vi "MF-101 I2C loopback dongle with command control and selectable output value.vi"() -> ()   [LabVIEW 8.6]
uses:
  <libdir>/resource/objmgr/ueidaq.rc
  vi.lib/UeiDaq/UeiDaqConfigureTimingForMessagingIO.vi
  vi.lib/UeiDaq/UeiDaqCreateI2CSlaveSession.vi
  vi.lib/UeiDaq/UeiDaqCreateI2CMasterSession.vi
panel:
  in  "Bus Monitor ACK":i32[](array[ring]) items=["Disabled", "Enabled"]
  in  "Bus Monitor":i32[](array[ring]) items=["Disabled", "Enabled"]
  in  "Termination":i32[](array[ring]) items=["Disabled", "Enabled"]
  in  "Loopback":i32[](array[ring]) items=["None", "Relay", "FPGA"]
  out "Bus Monitor ACK":i32[](array[ring]) items=["Disabled", "Enabled"]
  out "Bus Monitor":i32[](array[ring]) items=["Disabled", "Enabled"]
  out "Loopback":i32[](array[ring]) items=["None", "Relay", "FPGA"]
  out "AddressWidth":i32[](array[ring]) items=["7-bit", "10-bit"]
  in  "Slave Resource":string
  out "Termination":i32[](array[ring]) items=["750 Ohm", "1.5 kOhm"]
  in  "output value":u16
  in  "Message Size":i32
  out "Slave Read Data String":string
  out "Master Read Data String":string
  out "Slave Read Count":i32
  out "Master Read Count":i32
  in  "Command Type":u32(ring) items=["Write", "Read", "WriteRead"]
  out "Slave Tx Data":u16[](array[numeric]) format="%x"
  out "Slave Channel":i32
  out "Master Channel":i32
  in  "Stop":bool
  in  "Slave Address":i32
  in  "Slave Address Width":u32(ring) items=["7-bit", "10-bit"]
  in  "Bit Rate":i32(ring) items=["100kBitsPerSecond", "400kBitsPerSecond", "1MBitsPerSecond"]
  in  "TTL Level":i32(ring) items=["3.3V", "5V"]
  in  "Secure Shell?":bool
  out "Device Name":string
  in  "Master Resource":string
  # "I2C Loopback Example with static output value"
  # "Relay mode"
  # "dongle\n0-2, 2-0\n1-3, 3-1"
  # "Master and Slave\nCommon Configuration"
  # "Master Specific Configuration"
  # "Slave Specific Configuration"
  # "Device info"
  # "controls"
  # "indicators"
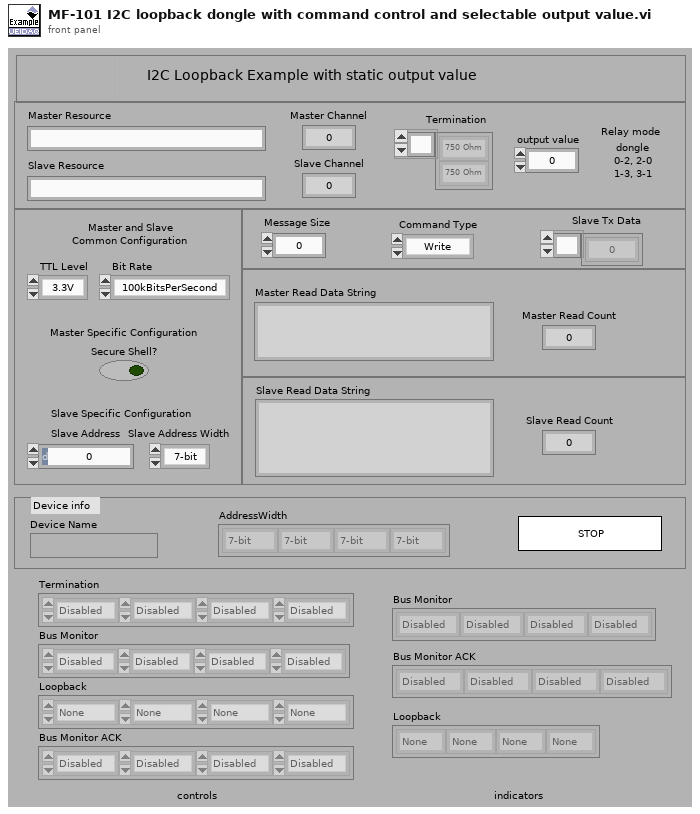
[diagram p1: front panel]
types:
  T1 = cluster{"Command":u32, "Slave Address":i32, "Slave Address Width":u32, "Number Elements to Write":i32, "Number Elements to Read":i32, "Write Data":u8[]}
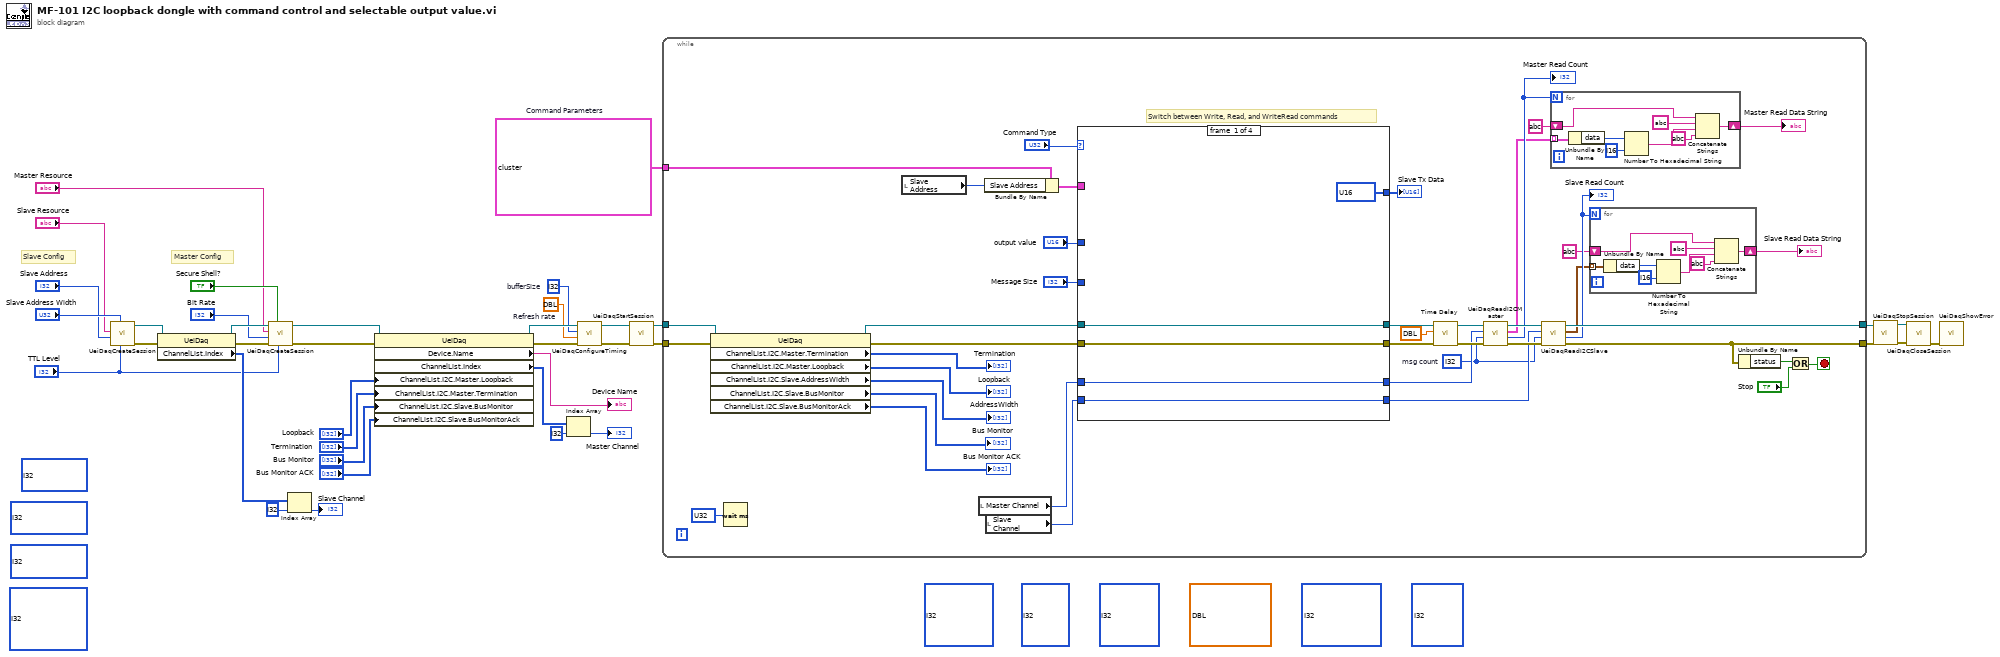
[diagram p0: block diagram]
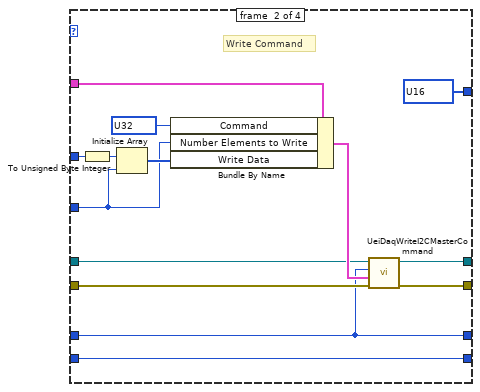
[diagram p2: hidden frame]
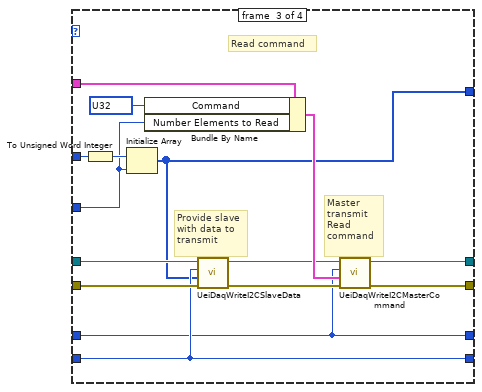
[diagram p3: hidden frame]
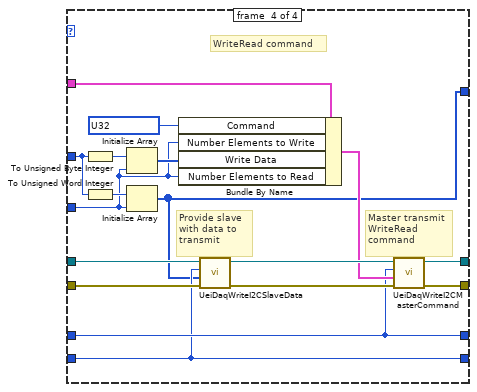
[diagram p4: hidden frame]
diagram:
  w1 = T1 ?  # Command Parameters
  (unwired) i32[] ? items=["Disabled", "Enabled"] ("Channel List:I2C:Slave:Bus Monitor ACK")
  (unwired) i32[] ? items=["Disabled", "Enabled"] ("Channel List:I2C:Slave:Bus Monitor")
  (unwired) i32[] ? ("Channel List:I2C:Slave:Address")
  (unwired) i32[] ? items=["7-bit", "10-bit"] ("Channel List:I2C:Slave:AddressWidth")
  (unwired) i32[] ? ("Channel List:I2C:Master:Byte to Byte Delay (us)")
  (unwired) i32[] ? items=["3.3V", "5V"] ("Channel List:I2C:TTL Level")
  (unwired) dbl[] ? ("Channel List:I2C:Custom Speed")
  (unwired) i32[] ? items=["100k BPS", "400k BPS", "1M BPS"] ("Channel List:I2C:Port Speed")
  (unwired) i32[] ? items=["Disabled", "Enabled"] ("Channel List:I2C:Master:Termination")
  w8 = dbl ?  # Refresh rate
  w9 = i32 ?  # bufferSize
  (unwired) i32[] ? items=["None", "Relay", "FPGA"] ("Channel List:I2C:Master:Loopback")
  # "Master Config"
  # "Slave Config"
  n1 = call-poly "UeiDaqCreateSession.vi"("TTL Level"="TTL Level", "Slave Address Width"="Slave Address Width", "Slave Address"="Slave Address", "Resource"="Slave Resource") -> ("error out"=w27:errorcluster, "UeiDaq Refnum Out"=w30:refnum<k20>)  [unwired: 6 in]
  n2 = property class="UeiDaq"(reference=w30, error in=w27) -> (reference out=w37:refnum<k20>, error out=w36:errorcluster, "ChannelList.Index"=w32:i32[])
  n3 = call-poly "UeiDaqCreateSession.vi"("TTL Level"="TTL Level", "Enable Secure Shell"="Secure Shell?", "error in (no error)"=w36, "Bit Rate"="Bit Rate", "Resource"="Master Resource", "UeiDaq Refnum In"=w37) -> ("error out"=w29:errorcluster, "UeiDaq Refnum Out"=w28:refnum<k20>)  [unwired: 4 in]
  n4 = Index Array(array=w32, index=i32 ?) -> (element=→"Slave Channel":i32)
  n5 = property class="UeiDaq"(reference=w28, error in=w29, "ChannelList.I2C.Master.Loopback"="Loopback", "ChannelList.I2C.Master.Termination"="Termination", "ChannelList.I2C.Slave.BusMonitor"="Bus Monitor", "ChannelList.I2C.Slave.BusMonitorAck"="Bus Monitor ACK") -> (reference out=w17:refnum<k20>, error out=w16:errorcluster, "Device.Name"=→"Device Name":string, "ChannelList.Index"=w31:i32[])
  n6 = Index Array(array=w31, index=i32 ?) -> (element=→"Master Channel":i32)
  n7 = call-poly "UeiDaqConfigureTiming.vi"("error in (no error)"=w16, "Refresh rate"=w8, "bufferSize"=w9, "UeiDaq Refnum In"=w17) -> ("error out"=w21:errorcluster, "UeiDaq Refnum Out"=w20:refnum<k20>)  [unwired: 6 in]
  n8 = call "UeiDaqStartSession.vi"("error in (no error)"=w21, "UeiDaq Refnum In"=w20) -> ("error out"=w19:errorcluster, "UeiDaq Refnum Out"=w18:refnum<k20>)  [unwired: 8 in]
  n9 = while {
    tunnel: w19 -> [w46]
    tunnel: w18 -> [w47]
    tunnel: [w74] -> w14
    tunnel: [w66] -> w13
    tunnel: w1 -> [w50]
    stop <- w54 stop-if-true
    w51 = i32 ?  # msg count
    # "Switch between Write, Read, and WriteRead commands"
    n10 = property class="UeiDaq"(reference=w47, error in=w46) -> (reference out=w43:refnum<k20>, error out=w45:errorcluster, "ChannelList.I2C.Master.Termination"=→"Termination":i32[], "ChannelList.I2C.Master.Loopback"=→"Loopback":i32[], "ChannelList.I2C.Slave.AddressWidth"=→"AddressWidth":i32[], "ChannelList.I2C.Slave.BusMonitor"=→"Bus Monitor":i32[], "ChannelList.I2C.Slave.BusMonitorAck"=→"Bus Monitor ACK":i32[])
    n11 = Wait (ms)(milliseconds to wait=u32 ?) -> ()  [unwired: 1 out]
    n12 = local read "Slave Address"() -> (w70:i32)
    n13 = local read "Master Channel"() -> (w55:i32)
    n14 = Bundle By Name(cluster=w50, "Slave Address"=w70) -> (w71:T1)
    n15 = local read "Slave Channel"() -> (w59:i32)
    n16 = case shown="2" "Command Type" {
      tunnel: w45 -> [w100 w109 w129 w143]
      tunnel: w43 -> [w96 w110 w128 w133]
      tunnel: "output value" -> [_ w112 w124 w144]
      tunnel: w71 -> [_ w103 w118 w142]
      tunnel: [w96 w101 w115 w140] -> w77
      tunnel: [w100 w108 w121 w139] -> w68
      tunnel: [u16[] ? u16[] ? w117 w131] -> w76
      tunnel: "Message Size" -> [_ w106 w116 w130]
      tunnel: w59 -> [w98 w105 w120 w134]
      tunnel: w55 -> [w97 w104 w119 w136]
      tunnel: [w98 w105 w120 w134] -> w58
      tunnel: [w97 w104 w119 w136] -> w57
      frame #0 {
      }
      frame #1 {
        w114 = u32 ? items=["Write", "Read", "WriteRead"] ("Command")
        # "Write Command"
        n17 = To Unsigned Byte Integer(number=w112) -> (unsigned 8bit integer=w102:u8)
        n18 = Initialize Array(w102, w106) -> (w113:u8[])
        n19 = Bundle By Name(cluster=w103, "Command"=w114, "Number Elements to Write"=w106, "Write Data"=w113) -> (w111:T1)
        n20 = call "UeiDaqWriteI2CMasterCommand.vi"("error in (no error)"=w109, "Command"=w111, "Port"=w104, "UeiDaq Refnum In"=w110) -> ("error out"=w108:errorcluster, "UeiDaq Refnum Out"=w101:refnum<k20>)  [unwired: 6 in]
      }
      frame #2 {
        w125 = u32 ? items=["Write", "Read", "WriteRead"] ("Command")
        # "Master \ntransmit\nRead\ncommand"
        # "Provide slave\nwith data to \ntransmit"
        # "Read command"
        n21 = To Unsigned Word Integer(number=w124) -> (unsigned 16bit integer=w123:u16)
        n22 = Initialize Array(w123, w116) -> (w117:u16[])
        n23 = Bundle By Name(cluster=w118, "Command"=w125, "Number Elements to Read"=w116) -> (w127:T1)
        n24 = call "UeiDaqWriteI2CSlaveData.vi"("error in (no error)"=w129, "Data"=w117, "Port"=w120, "UeiDaq Refnum In"=w128) -> ("error out"=w122:errorcluster, "UeiDaq Refnum Out"=w126:refnum<k20>)  [unwired: 5 in, 1 out]
        n25 = call "UeiDaqWriteI2CMasterCommand.vi"("error in (no error)"=w122, "Command"=w127, "Port"=w119, "UeiDaq Refnum In"=w126) -> ("error out"=w121:errorcluster, "UeiDaq Refnum Out"=w115:refnum<k20>)  [unwired: 6 in]
      }
      frame #3 {
        w132 = u32 ? items=["Write", "Read", "WriteRead"] ("Command")
        # "Master transmit\nWriteRead \ncommand"
        # "Provide slave \nwith data to\ntransmit"
        # "WriteRead command"
        n26 = To Unsigned Byte Integer(number=w144) -> (unsigned 8bit integer=w135:u8)
        n27 = To Unsigned Word Integer(number=w144) -> (unsigned 16bit integer=w145:u16)
        n28 = Initialize Array(w135, w130) -> (w146:u8[])
        n29 = Initialize Array(w145, w130) -> (w131:u16[])
        n30 = Bundle By Name(cluster=w142, "Command"=w132, "Number Elements to Write"=w130, "Write Data"=w146, "Number Elements to Read"=w130) -> (w137:T1)
        n31 = call "UeiDaqWriteI2CSlaveData.vi"("error in (no error)"=w143, "Data"=w131, "Port"=w134, "UeiDaq Refnum In"=w133) -> ("error out"=w138:errorcluster, "UeiDaq Refnum Out"=w141:refnum<k20>)  [unwired: 5 in, 1 out]
        n32 = call "UeiDaqWriteI2CMasterCommand.vi"("error in (no error)"=w138, "Command"=w137, "Port"=w136, "UeiDaq Refnum In"=w141) -> ("error out"=w139:errorcluster, "UeiDaq Refnum Out"=w140:refnum<k20>)  [unwired: 6 in]
      }
    }
    "Slave Tx Data" <- w76
    n33 = call "Time Delay"("error in (no error)"=w68, "Delay Time (s)"=dbl ?) -> ("error out"=w67:errorcluster)  [unwired: 9 in]
    n34 = call "UeiDaqReadI2CMaster.vi"("error in (no error)"=w67, "Message count"=w51, "Port"=w57, "UeiDaq Refnum In"=w77) -> ("error out"=w73:errorcluster, "return count"=w63:i32, "data"=w53:cluster{"stop bit":bool, "data":u8}[], "UeiDaq Refnum Out"=w75:refnum<k20>)  [unwired: 4 in]
    "Master Read Count" <- w63
    n35 = call "UeiDaqReadI2CSlave.vi"("error in (no error)"=w73, "Message count"=w51, "Port"=w58, "UeiDaq Refnum In"=w75) -> ("error out"=w66:errorcluster, "return count"=w61:i32, "data"=w52:cluster{"bus code":u32, "data":u8}[], "UeiDaq Refnum Out"=w74:refnum<k20>)  [unwired: 4 in]
    "Slave Read Count" <- w61
    n36 = for {
      N: w63 -> [_]
      shift-right: [w94] -> w65
      shift-left: string ? -> [w91]
      tunnel: w53 -> [w89] mode=indexing
      n37 = Unbundle By Name(w89) -> ("data"=w88:u8)
      n38 = Number To Hexadecimal String(1:i16 ? ("width (-)"), 2:w88) -> (0:w95:string)
      n39 = Concatenate Strings(w91, string ? ("string"), w95, string ? ("string")) -> (w94:string)
    }
    "Master Read Data String" <- w65
    n40 = for {
      N: w61 -> [_]
      tunnel: w52 -> [w81] mode=indexing
      shift-right: [w87] -> w62
      shift-left: string ? -> [w84]
      n41 = Unbundle By Name(w81) -> ("data"=w80:u8)
      n42 = Number To Hexadecimal String(1:i16 ? ("width (-)"), 2:w80) -> (0:w82:string)
      n43 = Concatenate Strings(w84, string ? ("string"), w82, string ? ("string")) -> (w87:string)
    }
    "Slave Read Data String" <- w62
    n44 = Unbundle By Name(w66) -> ("status"=w72:bool)
    n45 = Or(x=w72, y="Stop") -> (x .or. y?=w54:bool)
  }
  n46 = call "UeiDaqStopSession.vi"("error in (no error)"=w13, "UeiDaq Refnum In"=w14) -> ("error out"=w11:errorcluster, "UeiDaq Refnum Out"=w12:refnum<k20>)  [unwired: 8 in]
  n47 = call "UeiDaqCloseSession.vi"("error in (no error)"=w11, "UeiDaq Refnum In"=w12) -> ("error out"=w38:errorcluster)  [unwired: 1 in, 8 out]
  n48 = call "UeiDaqShowError.vi"("error in (no error)"=w38) -> ()  [unwired: 2 in, 9 out]
